vi "Práctica01_Ejercicio1_3.vi"() -> ()   [LabVIEW 2020]
panel:
  out "Array":dbl[](array[numeric])
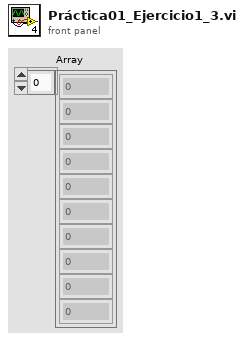
[diagram p1: front panel]
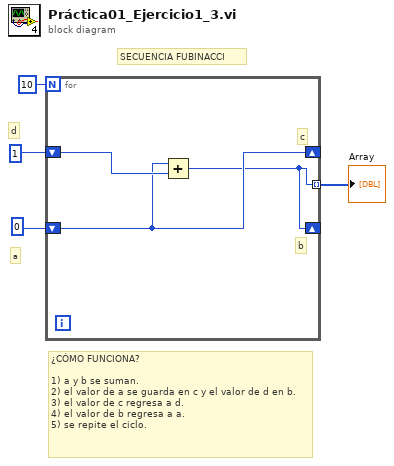
[diagram p0: block diagram]
diagram:
  # "SECUENCIA FUBINACCI"
  # "¿CÓMO FUNCIONA?\n\n1) a y b se suman.\n2) el valor de a se guarda en c y el valor de d en b.\n3) el valor de c regresa a d.\n4) el valor de b regresa a a.\n5) se repite el ciclo."
  # "d"
  # "a"
  n1 = for {
    N: 10 -> [_]
    shift-right: [w5] -> _
    shift-left: 0 -> [w6]
    shift-right: [w6] -> _
    shift-left: 1 -> [w7]
    tunnel: [w5] -> w1 mode=indexing
    # "c"
    # "b"
    n2 = Add(x=w6, y=w7) -> (x+y=w5:i32)
  }
  "Array" <- w1
